vi "Keysight E36300 Series Output Trigger Level.vi"() -> ()   [LabVIEW 2020]
doc: "This example shows how to configure the trigger level."
uses:
  Keysight E36300 Series.lvlib
panel:
  in  "Current Level (2 A)":dbl=0.001
  in  "Voltage Level (1 V)":dbl=0.001
  in  "Channel (1)":string="1"
  out "Actual Voltage Level (V)":dbl[](array[numeric]) format="%.3g"
  out "Actual Current Level (A)":dbl[](array[numeric]) format="%.3g"
  in  "VISA resource name":refnum<visa-resource-name>
  # "(c) 2019 - 2021 National Instruments.  ALL RIGHTS RESERVED."
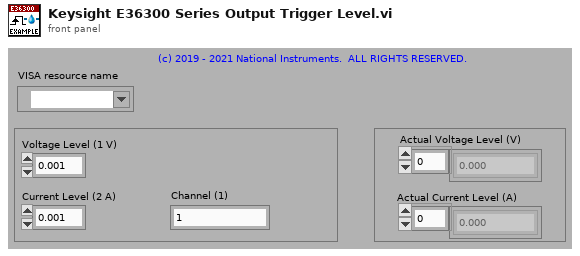
[diagram p1: front panel]
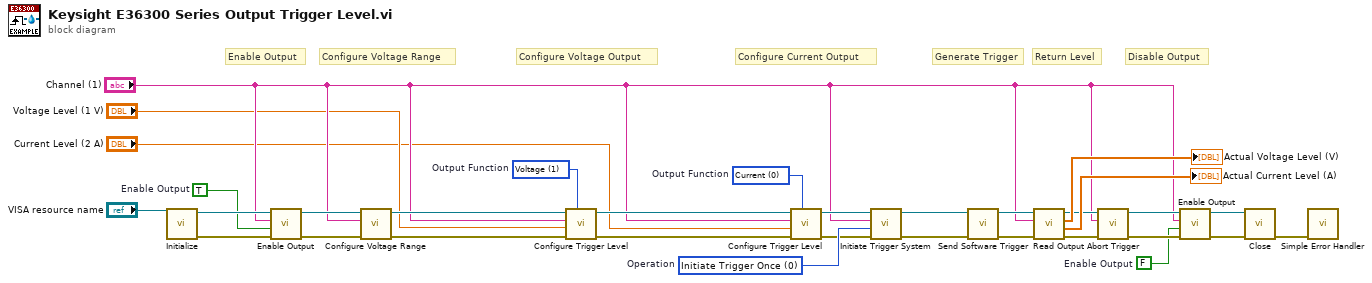
[diagram p0: block diagram]
diagram:
  w3 = FALSE  # Enable Output
  w9 = u16 0 items=["Initiate Trigger Once", "Initiate Trigger Continuously", "Stop Continuously Trigger"]  # Operation
  w24 = TRUE  # Enable Output
  w28 = 0 items=["Current", "Voltage"]  # Output Function
  w8 = 1 items=["Current", "Voltage"]  # Output Function
  # "Generate Trigger"
  # "Disable Output"
  # "Enable Output"
  # "Configure Current Output"
  # "Configure Voltage Output"
  # "Return Level"
  # "Configure Voltage Range"
  n1 = call "Initialize.vi"("VISA resource name"="VISA resource name") -> ("error out"=w25:errorcluster, "VISA resource name out"=w26:refnum<visa-resource-name>)  [unwired: 9 in]
  n2 = call "Enable Output.vi"("error in (no error)"=w25, "Enable Output (F: Disable)"=w24, "Channel (1)"="Channel (1)", "VISA resource name"=w26) -> ("error out"=w7:errorcluster, "VISA resource name out"=w23:refnum<visa-resource-name>)  [unwired: 6 in]
  n3 = call "Configure Voltage Range.vi"("error in (no error)"=w7, "Channel (1)"="Channel (1)", "VISA resource name"=w23) -> ("error out"=w15:errorcluster, "VISA resource name out"=w16:refnum<visa-resource-name>)  [unwired: 7 in]
  n4 = call "Configure Trigger Level.vi"("Output Function (0: Voltage)"=w8, "error in (no error)"=w15, "Trigger Level (0.001)"="Voltage Level (1 V)", "Channel (1)"="Channel (1)", "VISA resource name"=w16) -> ("error out"=w6:errorcluster, "VISA resource name out"=w27:refnum<visa-resource-name>)  [unwired: 5 in]
  n5 = call "Configure Trigger Level.vi"("Output Function (0: Voltage)"=w28, "error in (no error)"=w6, "Trigger Level (0.001)"="Current Level (2 A)", "Channel (1)"="Channel (1)", "VISA resource name"=w27) -> ("error out"=w4:errorcluster, "VISA resource name out"=w10:refnum<visa-resource-name>)  [unwired: 5 in]
  n6 = call "Initiate Trigger System.vi"("error in (no error)"=w4, "Operation (0 : Initiate Trigger Once)"=w9, "Channel (1)"="Channel (1)", "VISA resource name"=w10) -> ("error out"=w13:errorcluster, "VISA resource name out"=w14:refnum<visa-resource-name>)  [unwired: 6 in]
  n7 = call "Send Software Trigger.vi"("error in (no error)"=w13, "VISA resource name"=w14) -> ("error out"=w11:errorcluster, "VISA resource name out"=w12:refnum<visa-resource-name>)  [unwired: 8 in]
  n8 = call "Read Output.vi"("error in (no error)"=w11, "Channel (1)"="Channel (1)", "VISA resource name"=w12) -> ("error out"=w18:errorcluster, "Actual Current Level (A)"=→"Actual Current Level (A)":dbl[], "Actual Voltage Level (V)"=→"Actual Voltage Level (V)":dbl[], "VISA resource name out"=w20:refnum<visa-resource-name>)  [unwired: 5 in]
  n9 = call "Abort Trigger.vi"("error in (no error)"=w18, "Channel (1)"="Channel (1)", "VISA resource name"=w20) -> ("error out"=w17:errorcluster, "VISA resource name out"=w19:refnum<visa-resource-name>)  [unwired: 7 in]
  n10 = call "Enable Output.vi"("error in (no error)"=w17, "Enable Output (F: Disable)"=w3, "Channel (1)"="Channel (1)", "VISA resource name"=w19) -> ("error out"=w21:errorcluster, "VISA resource name out"=w22:refnum<visa-resource-name>)  [unwired: 6 in]
  n11 = call "Close.vi"("error in (no error)"=w21, "VISA resource name"=w22) -> ("error out"=w29:errorcluster)  [unwired: 9 in]
  n12 = call <vilib>:"Simple Error Handler.vi"("error in (no error)"=w29) -> ()  [unwired: 4 in, 5 out]
